vi "Queue Last Ack.vi"(10 "Queue Actor":refnum<class "Queue Actor.lvclass">, 11 "jettl Queue Actor in":refnum<class "jettl Queue Actor.lvclass">) -> (3 "jettl Queue Actor out":refnum<class "jettl Queue Actor.lvclass">)   [LabVIEW 2021, in "jettl.lvlib" / "jettl Queue Actor.lvclass"]
uses:
  jettl Queue Actor.lvclass
  Actor/Queue Actor/Queue Actor.lvclass
  jettl Queue Actor.lvclass/jettl Queue Actor.ctl
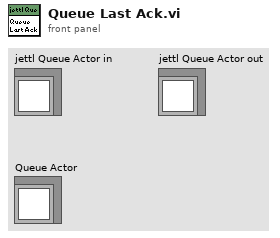
[diagram p1: front panel]
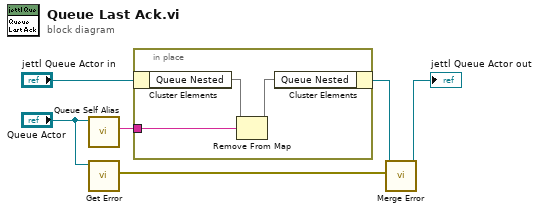
[diagram p0: block diagram]
diagram:
  n1 = call-dynamic "Queue Self Alias.vi"("Actor in"="Queue Actor") -> ("Queue Self Alias"=w5:string)  [unwired: 10 in]
  n2 = call-dynamic "Get Error.vi"("Actor in"="Queue Actor") -> ("Error"=w4:errorcluster)  [unwired: 10 in]
  n3 = in-place {
    in-place-border: w5 -> [w7]
    n4 = in-place-cluster #1("jettl Queue Actor in") -> ("Queue Nested"=w8:map{string, refnum<data-value>})
    n5 = Remove From Map(10:w7, 11:w8) -> (3:w9:map{string, refnum<data-value>})  [unwired: 2 out]
    n6 = in-place-cluster #1("Queue Nested"=w9) -> (w3:refnum<class "jettl Queue Actor.lvclass">)
  }
  n7 = call-dynamic "Merge Error.vi"("Error"=w4, "jettl Queue Actor in"=w3) -> ("jettl Queue Actor out"=→"jettl Queue Actor out":refnum<class "jettl Queue Actor.lvclass">)  [unwired: 9 in]
